vi "Update History.vi"(8 "error in (no error)":errorcluster, 10 "Optimisation result":T1, 11 "Run Optimiser in":refnum<class "Optimiser Cell.lvclass">) -> (0 "error out":errorcluster, 3 "Run Optimiser out":refnum<class "Optimiser Cell.lvclass">)   [LabVIEW 2020, in "Run Utilities.lvlib" / "Optimiser Cell.lvclass"]
uses:
  Optimiser Cell.lvclass
  Optimiser Results.ctl
  Name with value pair.ctl
  Optimiser Cell.lvclass/Optimiser Cell.ctl
  Classes/Log/Log.lvclass/Log.ctl
  Ancestor/Ancestor/Ancestor.lvclass/Ancestor.ctl
  Classes/Log/Write.vi
  Support VIs/Generate Error.vi
  Support VIs/Date n Time.vi
  FGV/Error Memory/Get Error Description.vi
  Support VIs/Get PC name.vi
  Ancestor/Ancestor/Read ID.vi
  Support VIs/Get Class Name.vi
  <vilib>/Utility/error.llb/Clear Errors.vi
  FGV/Error Memory/Error Memory Core.vi
  <vilib>/AdvancedString/Delimited String to 1D String Array.vi
  Support VIs/Circus Root Path.vi
  FGV/Error Memory/Error Crt Lvl checker.vi
  FGV/Error Memory/Error Memory Core.vi/40c8088d-b597-4017-91af-faa98e00292e.vi
  FGV/Error Memory/Error Memory Core.vi/d4a3ab98-063c-4e44-b43d-fbdcfe6c2be2.vi
  Classes/Log/Rotate.vi
  Support VIs/Global Memory.vi
  <vilib>/Utility/LVClass/Get LV Class Name.vi
  Support VIs/Is in Packed Library.vi
  Support VIs/TALOS Root path.vi
  Support VIs/Read CSV worksheet.vi
  Support VIs/Global Constants.vi
  <vilib>/Utility/error.llb/General Error Handler.vi
  Ancestor/Ancestor/Ancestor.lvclass
  <vilib>/Comparison/Equal/Equal Functor/Equal Functor.lvclass
  Interfaces/Analysis Framework/Analysis Framework.lvclass
  Classes/Log/Log.lvclass
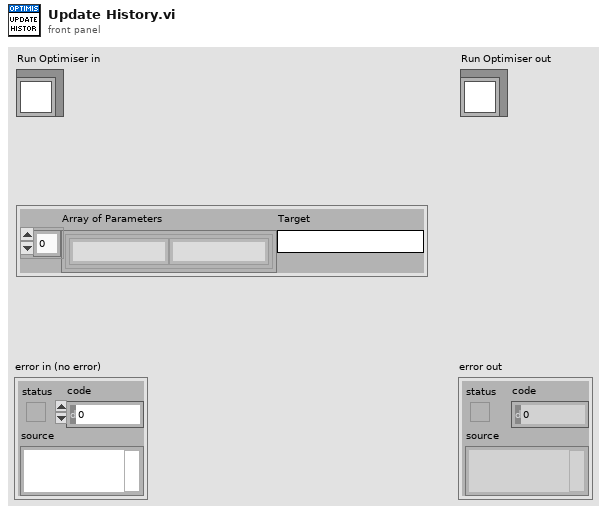
[diagram p1: front panel]
types:
  T1 = typedef "Run Utilities.lvlib/Optimiser Cell.lvclass/Optimiser Results.ctl" = cluster{"Array of Parameters":T2[], "Target":string}
  T2 = typedef "Analysis Framework.lvclass/Name with value pair.ctl" = cluster{"Name":string, "Value":string}
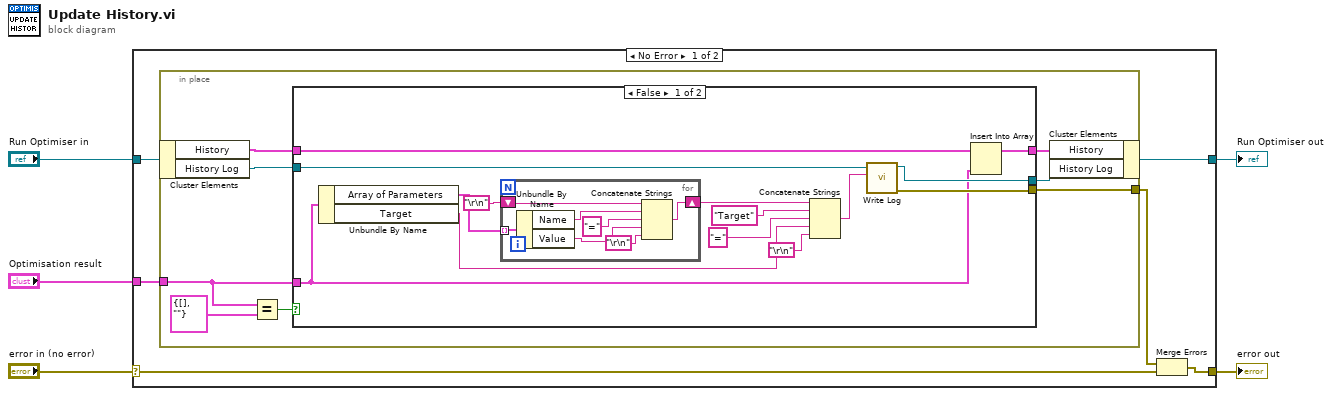
[diagram p0: block diagram]
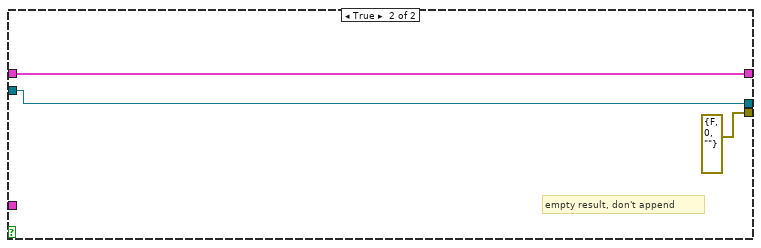
[diagram p2: hidden frame]
diagram:
  n1 = case shown="No Error" "error in (no error)" {
    selector: "error in (no error)" -> [w7 w45]
    tunnel: [w6 w45] -> w4
    tunnel: [w11 w44] -> w2
    tunnel: "Run Optimiser in" -> [w9 w44]
    tunnel: "Optimisation result" -> [w10 _]
    frame No Error {
      n2 = in-place {
        in-place-border: w10 -> [w15]
        in-place-border: [w12] -> w8
        n3 = in-place-cluster #1(w9) -> ("History"=w19:T1[], "History Log"=w14:refnum<class "Log.lvclass">)
        n4 = Equal?(x=w15, y=T1 {"Array of Parameters"=[], "Target"=""} ("x")) -> (x = y?=w17:bool)
        n5 = case shown="False" w17 {
          tunnel: w19 -> [w33 w43]
          tunnel: [w32 w43] -> w18
          tunnel: w15 -> [w28 _]
          tunnel: w14 -> [w31 w42]
          tunnel: [w30 w42] -> w13
          tunnel: [w29 errorcluster {"status"=FALSE, "code"=0, "source"=""} ("error out")] -> w12
          frame False {
            n6 = Unbundle By Name(w28) -> ("Array of Parameters"=w27:T2[], "Target"=w22:string)
            n7 = for {
              shift-right: [w35] -> w26
              shift-left: "\r\n" -> [w40]
              tunnel: w27 -> [w39] mode=indexing
              n8 = Unbundle By Name(w39) -> ("Name"=w38:string, "Value"=w36:string)
              n9 = Concatenate Strings(w40, w38, "=" ("delimiter"), w36, "\r\n") -> (w35:string)
            }
            n10 = Concatenate Strings(w26, "Target" ("string"), "=" ("string"), w22, "\r\n") -> (w21:string)
            n11 = call "Write Log.vi"("Text"=w21, "Log in"=w31) -> ("error out"=w29:errorcluster, "Log out"=w30:refnum<class "Log.lvclass">)  [unwired: 8 in]
            n12 = Insert Into Array(array=w33, new element=w28) -> (w32:T1[])  [unwired: 1 in]
          }
          frame True {
            # "empty result, don't append"
          }
        }
        n13 = in-place-cluster #1("History"=w18, "History Log"=w13) -> (w11:refnum<class "Optimiser Cell.lvclass">)
      }
      n14 = Merge Errors(w8, w7) -> (w6:errorcluster)
    }
    frame Error {
    }
  }
  "error out" <- w4
  "Run Optimiser out" <- w2
